vi "Coord window-Load.vi"(11 "selected path":path) -> (0 "error out":errorcluster)   [LabVIEW 2013]
uses:
  Program Files (x86)/National Instruments/LabVIEW 2013/user.lib/My Palettes.lib/Files & paths/Spreadsheet/Read From Spreadsheet File (string)-Mod.vi
  Globals/Coord window-Globals.vi
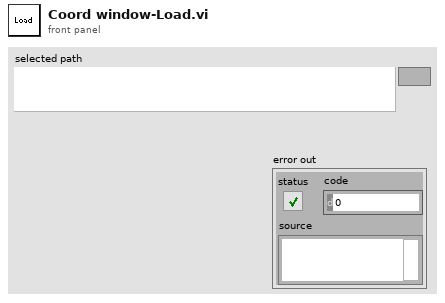
[diagram p1: front panel]
types:
  T1 = typedef "Coordinate list window refs.ctl" = cluster{"Window Name (i.e. Key)":string, "menu reference":refnum<k9>, "VI's reference":refnum<vi>, "Pane 1":refnum<vi>, "Pane 2":refnum<vi>, "Coord Listbox":refnum<vi>, "File name":refnum<vi>, "Picture Map":refnum<vi>, "Stage XYZ Position ind.":refnum<vi>}
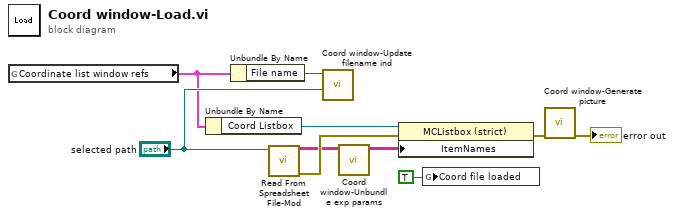
[diagram p0: block diagram]
diagram:
  n1 = global read "Coord window-Globals.vi" "Coordinate list window refs"() -> (w4:T1)
  n2 = Unbundle By Name(w4) -> ("Coord Listbox"=w8:refnum<vi>)
  n3 = Unbundle By Name(w4) -> ("File name"=w9:refnum<vi>)
  n4 = call-poly "Read From Spreadsheet File-Mod.vi"("file path (dialog if empty)"="selected path") -> ("all rows"=w3:string[][], "error out"=w7:errorcluster)  [unwired: 9 in, 4 out]
  n5 = call "Coord window-Update filename ind.vi"("File path"="selected path", "File name indicator ref"=w9) -> ()  [unwired: 9 in, 1 out]
  n6 = call "Coord window-Unbundle exp params.vi"("Item Names + exp params"=w3) -> ("Item Names"=w2:string[][])  [unwired: 10 in]
  n7 = property on="Property Node" class="MCListbox (strict)"(reference=w8, error in=w7, "ItemNames"=w2) -> (error out=w6:errorcluster)  [unwired: 1 out]
  n8 = global write "Coord window-Globals.vi" "Coord file loaded"(TRUE ("Initialised")) -> ()
  n9 = call "Coord window-Generate picture.vi"("error in (no error)"=w6) -> ("error out"=→"error out":errorcluster)  [unwired: 10 in]
